vi "FPGAcode4_SmallArray.vi"() -> ()   [LabVIEW 2015]
uses:
  Limits_In.ctl
  Detector_Cluster.ctl
  <vilib>/Platform/TimedLoop/XDataNode/timing_clust.ctl
  <vilib>/Platform/TimedLoop/XDataNode/nitl_modes.ctl
  <vilib>/Platform/TimedLoop/XDataNode/wakeup.ctl
  Correlations.ctl
  <vilib>/rvi/Emulation/niFpgaSctlEmulationGetInTimedLoop.vi
  <vilib>/rvi/Emulation/niFpgaEmulationReportErrorSimple.vi
  <vilib>/rvi/Emulation/niFpgaGetClockAttributes.vi
  <vilib>/rvi/Emulation/niFpgaCriticalErrorInLSC.vi
  <vilib>/rvi/eio/common/nirviEmuTemplateMethod_errors.vi
  <vilib>/rvi/Emulation/niFpgaEmulationIsFPGAContextNoSignature.vi
  <vilib>/rvi/DataTransferAndStorage/Container/Common/niFpgaContainerGetUniqueNameForEmu.vi
  <vilib>/rvi/eio/common/nirviEmuReportErrorAndStop.vi
  <vilib>/rvi/Emulation/niFpgaProcessEmulError.vi
  <vilib>/Platform/TimedLoop/XDataNode/XDataNode.xnode
  <vilib>/eio/EIONode/EIONode.xnode
  <vilib>/rvi/DataTransferAndStorage/Container/XNode/niFpgaContainer.xnode
  <vilib>/rvi/DataTransferAndStorage/Handshake/Emulation/niFpgaHandshakeEmulation.vi
  <vilib>/Platform/TimedLoop/XDataNode/XDNodeRunTimeDep.lvlib
panel:
  in  "Charge Error Factor":fxp<+,32,0>=0.19999999995343387 format="%_2g"
  in  "Calibrate":bool=TRUE
  in  "Limits":T1={"High Charge Limit"=4.54747350780585e-13, "Low Charge Limit"=0.0, "High Velocity Limit"=262143.0, "Low Velocity Limit"=0.0, "High Mass Limit"=7.27595761248936e-12, "Low Mass Limit"=0.0, "High Voltage"=2200000.0}
  in  "One Shot":bool
  in  "Threshold Factor":fxp<+/-,32,16>=1.149993896484375 format="%.2g"
  in  "Armed":bool
  in  "User Trigger Distance":fxp<+/-,34,18> format="%.3g"
  in  "User Trigger?":bool
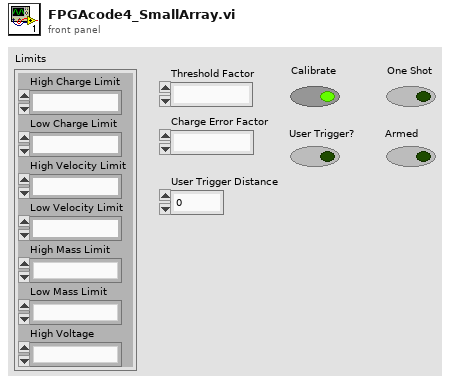
[diagram p1: front panel]
types:
  T1 = typedef "Limits_In.ctl" = cluster{"High Charge Limit":fxp<+,32,-41>, "Low Charge Limit":fxp<+,32,-41>, "High Velocity Limit":fxp<+,18,18>, "Low Velocity Limit":fxp<+,18,18>, "High Mass Limit":fxp<+,32,-37>, "Low Mass Limit":fxp<+,32,-37>, "High Voltage":fxp<+,32,22>}
  T2 = cluster{"[0]":fxp<+,16,1>, "[1]":fxp<+,16,1>, "[2]":fxp<+,16,1>, "[3]":fxp<+,16,1>, "[4]":fxp<+,16,1>, "[5]":fxp<+,16,1>, "[6]":fxp<+,16,1>, "[7]":fxp<+,16,1>, "[8]":fxp<+,16,1>, "[9]":fxp<+,16,1>, "[10]":fxp<+,16,1>}
  T3 = cluster{"[0]":i32, "[1]":i32, "[2]":i32, "[3]":i32, "[4]":i32, "[5]":i32, "[6]":i32, "[7]":i32, "[8]":i32, "[9]":i32, "[10]":i32}
  T4 = cluster{"[0]":cluster{"Detector Max Speed Count":i32, "Detector Min Speed Count":i32, "Gap Max Speed Count":i32, "Gap Min Speed Count":i32}, "[1]":cluster{"Detector Max Speed Count":i32, "Detector Min Speed Count":i32, "Gap Max Speed Count":i32, "Gap Min Speed Count":i32}, "[2]":cluster{"Detector Max Speed Count":i32, "Detector Min Speed Count":i32, "Gap Max Speed Count":i32, "Gap Min Speed Count":i32}, "[3]":cluster{"Detector Max Speed Count":i32, "Detector Min Speed Count":i32, "Gap Max Speed Count":i32, "Gap Min Speed Count":i32}, "[4]":cluster{"Detector Max Speed Count":i32, "Detector Min Speed Count":i32, "Gap Max Speed Count":i32, "Gap Min Speed Count":i32}, "[5]":cluster{"Detector Max Speed Count":i32, "Detector Min Speed Count":i32, "Gap Max Speed Count":i32, "Gap Min Speed Count":i32}, "[6]":cluster{"Detector Max Speed Count":i32, "Detector Min Speed Count":i32, "Gap Max Speed Count":i32, "Gap Min Speed Count":i32}, "[7]":cluster{"Detector Max Speed Count":i32, "Detector Min Speed Count":i32, "Gap Max Speed Count":i32, "Gap Min Speed Count":i32}, "[8]":cluster{"Detector Max Speed Count":i32, "Detector Min Speed Count":i32, "Gap Max Speed Count":i32, "Gap Min Speed Count":i32}, "[9]":cluster{"Detector Max Speed Count":i32, "Detector Min Speed Count":i32, "Gap Max Speed Count":i32, "Gap Min Speed Count":i32}, "[10]":cluster{"Detector Max Speed Count":i32, "Detector Min Speed Count":i32, "Gap Max Speed Count":i32, "Gap Min Speed Count":i32}}
  T5 = cluster{cluster{"[0]":i32, "[1]":i32, "[2]":i32, "[3]":i32, "[4]":i32, "[5]":i32, "[6]":i32, "[7]":i32, "[8]":i32, "[9]":i32, "[10]":i32}, cluster{"[0]":i32, "[1]":i32, "[2]":i32, "[3]":i32, "[4]":i32, "[5]":i32, "[6]":i32, "[7]":i32, "[8]":i32, "[9]":i32, "[10]":i32}, cluster{"[0]":i32, "[1]":i32, "[2]":i32, "[3]":i32, "[4]":i32, "[5]":i32, "[6]":i32, "[7]":i32, "[8]":i32, "[9]":i32, "[10]":i32}, cluster{"[0]":i32, "[1]":i32, "[2]":i32, "[3]":i32, "[4]":i32, "[5]":i32, "[6]":i32, "[7]":i32, "[8]":i32, "[9]":i32, "[10]":i32}}
  T6 = cluster{"Distance to PSU":fxp<+/-,64,37>, "Distance to end of PSU":fxp<+/-,64,37>, "Distance to DCS 2":fxp<+/-,64,37>, "Distance to DCS 1":fxp<+/-,64,37>, "Distance to front of LEIL Chamber":fxp<+/-,64,37>}
  T7 = typedef "Detector_Cluster.ctl" = cluster{"Det 1":i32, "Det 2":i32}
  T8 = cluster{"Filter 1":T7, "Filter 2":T7, "Filter 3":T7, "Filter 4":T7}
  T9 = cluster{"Detector Max Speed Count":i32, "Detector Min Speed Count":i32, "Gap Max Speed Count":i32, "Gap Min Speed Count":i32}[]
  T10 = cluster{"Filter 1":T7, "Filter 2":T7, "Filter 3":T7, "Filter 4":T7}[]
  T11 = typedef "XDNodeRunTimeDep.lvlib/timing_clust.ctl" = cluster{"Expected End [f-1]":u64, "Actual End [f-1]":u64, "Finished Late? [f-1]":bool, "Expected End [i-1]":u64, "Actual End [i-1]":u64, "Finished Late? [i-1]":bool, "Expected Start [i]":u64, "Actual Start [i]":u64, "Expected Start [f]":u64, "Actual Start [f]":u64, "Source Name":string, "Structure Name":string, "Period":i64, "Deadline":i64, "Offset":i64, "Start":i64, "Priority":i32, "Timeout":i32, "Mode":T12, "Wakeup Reason":T13, "Error":errorcluster, "Source Type":string, "Secondary Source Type":string, "Global End Time":u64, "Global Start Time":u64, "Frame Duration":u64, "Iteration Duration":u64, "Assigned CPU":i32, "I/O Scan Engine Mode":u32}
  T12 = typedef "XDNodeRunTimeDep.lvlib/nitl_modes.ctl" = enum32{"No Change", "Process missed periods, maintain original phase", "Discard missed periods, maintain original phase", "Process missed periods, ignore original phase", "Discard missed periods, ignore original phase"}
  T13 = typedef "XDNodeRunTimeDep.lvlib/wakeup.ctl" = enum32{"Normal", "Aborted", "Asynchronous wakeup", "Timing source error", "Timed loop error", "Timeout"}
  T14 = cluster{"IO Module\\AI 0":i16, "IO Module\\AI 1":i16}
  T15 = cluster{"First Detector Count":i32, "Detector Gap Count":i32, "Second Detector Count":i32, "Second Detector Final Count":i32}
  T16 = typedef "Correlations.ctl" = cluster{"First Correlation":i32, "Latest Correlation":i32}
  T17 = cluster{"Data":fxp<+/-,40,32>, "Data":fxp<+/-,40,32>}
  T18 = cluster{cluster{"Data":i16, "Data":i16}, cluster{"Det 1":i16, "Det 2":i16}, cluster{"Det 1":i16, "Det 2":i16}, cluster{"Det 1":i16, "Det 2":i16}}
  T19 = cluster{cluster{"Det 1":i16, "Det 2":i16}, cluster{"Det 1":i16, "Det 2":i16}, cluster{"Det 1":i16, "Det 2":i16}, cluster{"Det 1":i16, "Det 2":i16}}
  T20 = cluster{"Distance to PSU":fxp<+/-,64,69>, "Distance to end of PSU":fxp<+/-,64,69>, "Distance to DCS 2":fxp<+/-,64,69>, "Distance to DCS 1":fxp<+/-,64,69>, "Distance to front of LEIL Chamber":fxp<+/-,64,69>}
  T21 = cluster{"Distance to PSU":i32, "Distance to end of PSU":i32, "Distance to DCS 2":i32, "Distance to DCS 1":i32, "Distance to front of LEIL Chamber":i32}
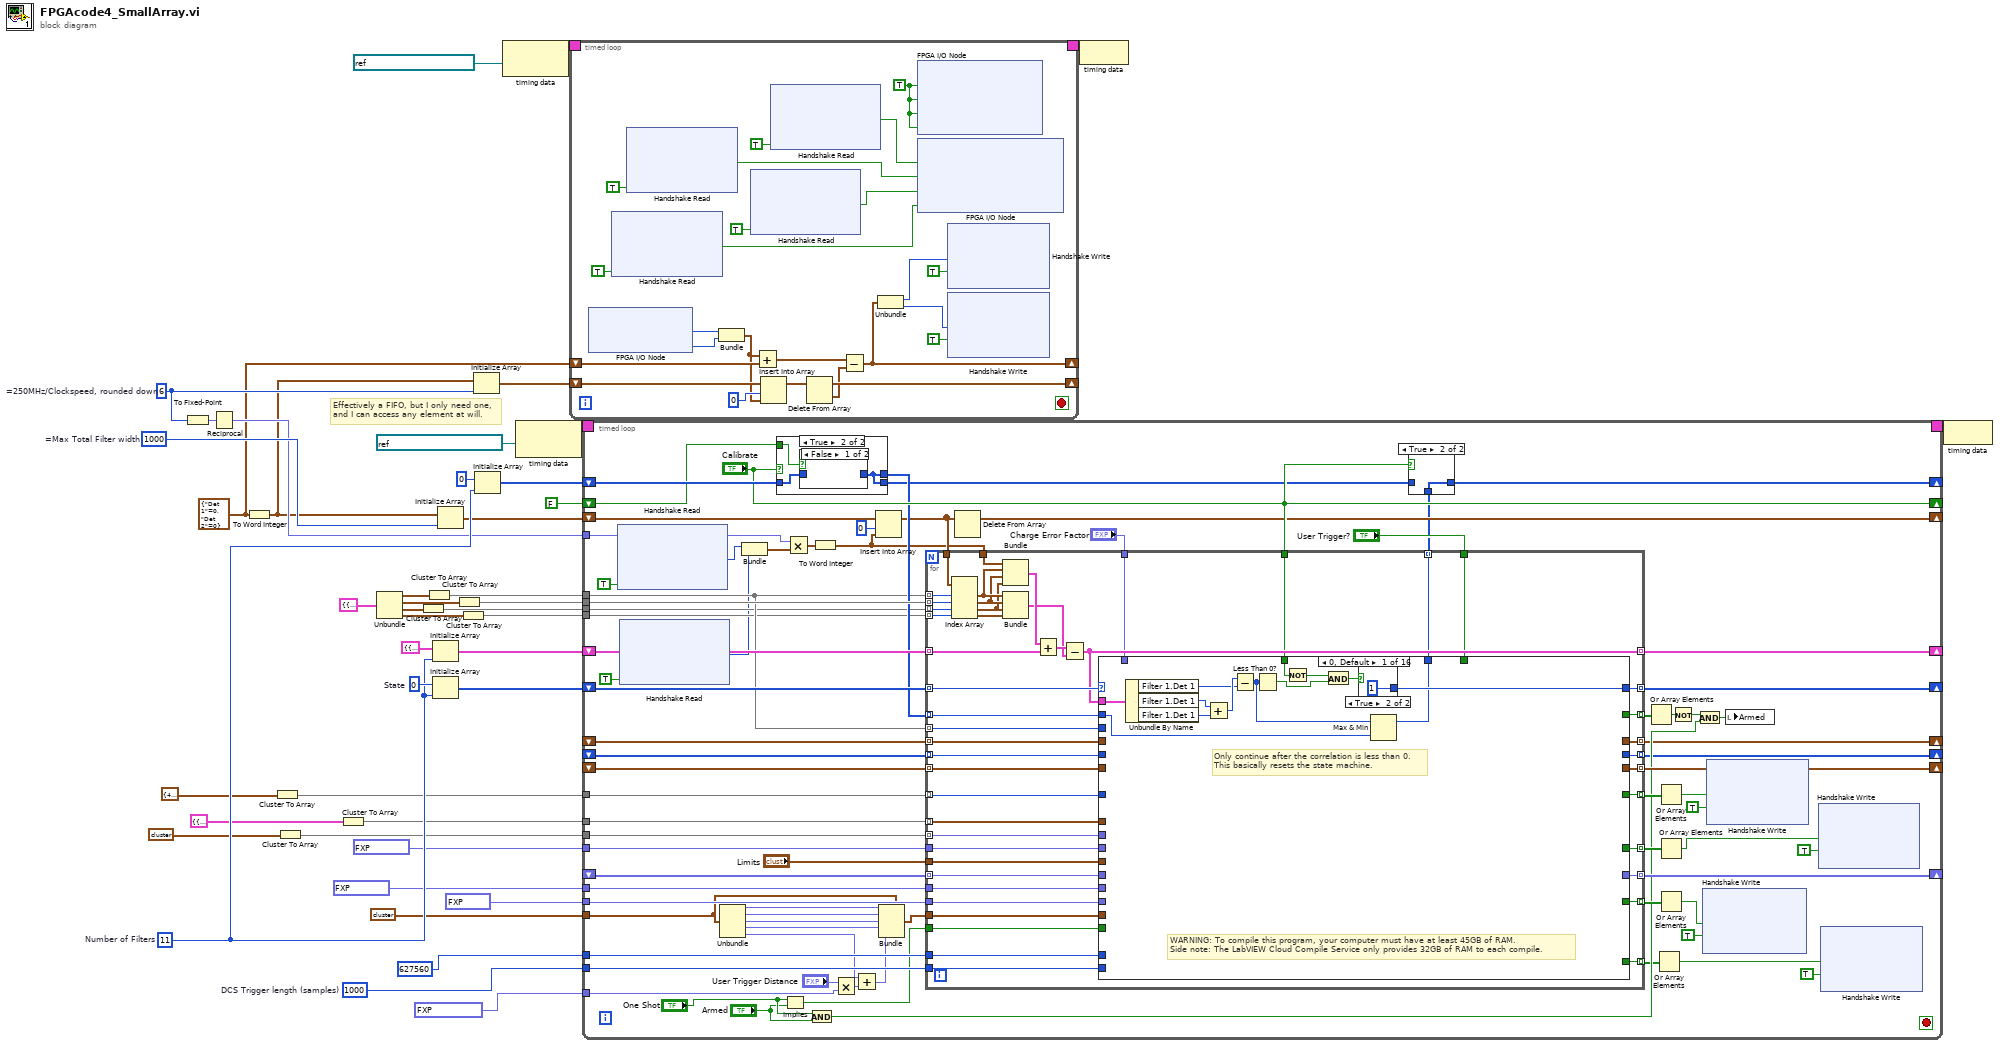
[diagram p0: block diagram]
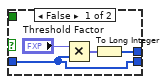
[diagram p2: hidden frame]
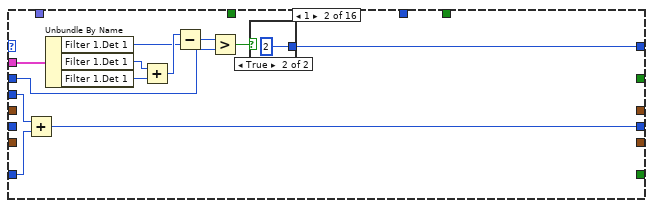
[diagram p6: hidden frame]
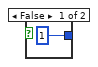
[diagram p7: hidden frame]
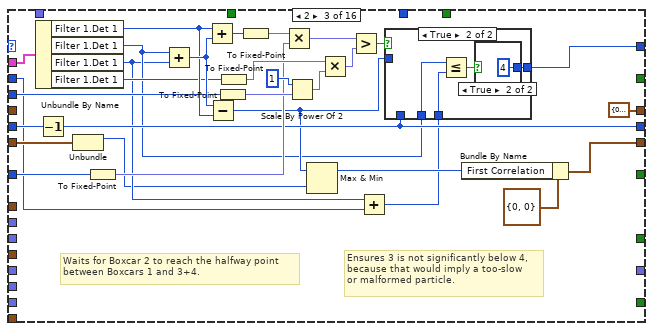
[diagram p8: hidden frame]
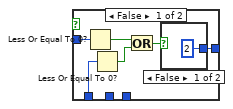
[diagram p9: hidden frame]
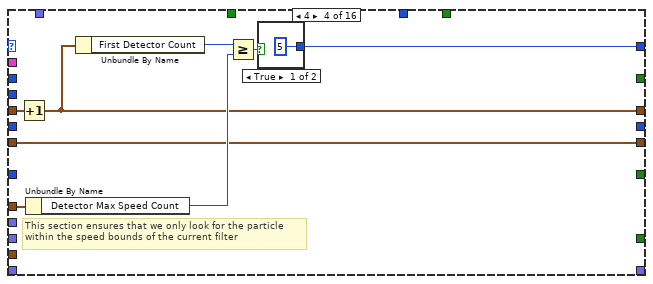
[diagram p12: hidden frame]
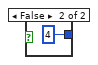
[diagram p13: hidden frame]
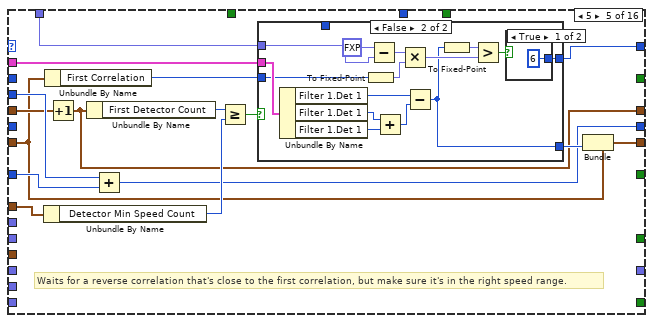
[diagram p14: hidden frame]
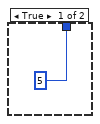
[diagram p15: hidden frame]
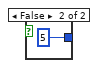
[diagram p16: hidden frame]
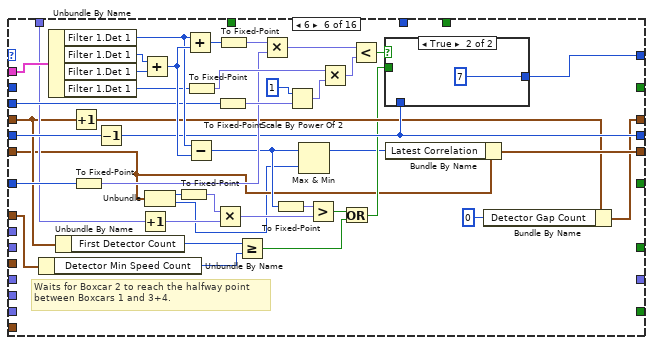
[diagram p17: hidden frame]
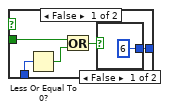
[diagram p18: hidden frame]
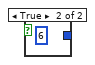
[diagram p19: hidden frame]
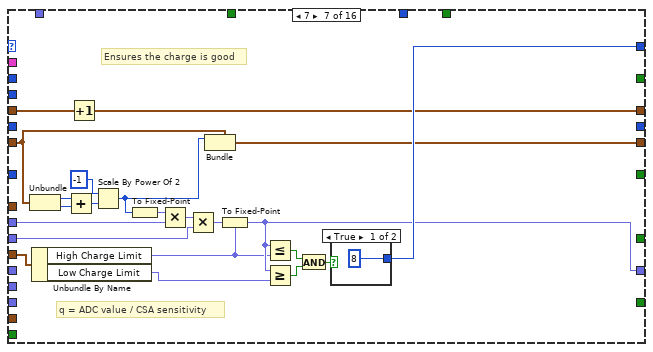
[diagram p20: hidden frame]
diagram:
  w35 = u8 6  # =250MHz/Clockspeed, rounded down
  w40 = 1000  # =Max Total Filter width
  w5 = u16 1000  # DCS Trigger length (samples)
  w2 = T7 {"Det 1"=0, "Det 2"=0} ("Detectors")
  w44 = u8 0  # State
  w41 = 11  # Number of Filters
  # "Effectively a FIFO, but I only need one,\nand I can access any element at will."
  n1 = To Fixed-Point(number=w35) -> (fixed-point=w37:fxp<+,8,8>)  [unwired: 1 in]
  n2 = Reciprocal(x=w37) -> (1/x=w20:fxp<+,9,1>)
  n3 = To Word Integer(number=w2) -> (16bit integer=w1:cluster{"Det 1":i16, "Det 2":i16})
  n4 = Cluster To Array(cluster=T3 {"[0]"=4000, "[1]"=2359, "[2]"=1391, "[3]"=820, "[4]"=484, "[5]"=285, "[6]"=168, "[7]"=99, "[8]"=59, "[9]"=35, "[10]"=20}) -> (array=w13:i32[])
  n5 = Cluster To Array(cluster=T2 {"[0]"=0.000823974609375, "[1]"=0.000823974609375, "[2]"=0.000823974609375, "[3]"=0.000823974609375, "[4]"=0.000823974609375, "[5]"=0.00152587890625, "[6]"=0.003265380859375, "[7]"=0.007080078125, "[8]"=0.015869140625, "[9]"=0.03704833984375, "[10]"=0.100006103515625} ("cluster 3")) -> (array=w11:fxp<+,16,1>[])
  n6 = Cluster To Array(cluster=T4 {"[0]"={"Detector Max Speed Count"=42000, "Detector Min Speed Count"=84000, "Gap Max Speed Count"=78000, "Gap Min Speed Count"=156000}, "[1]"={"Detector Max Speed Count"=21477, "Detector Min Speed Count"=42953, "Gap Max Speed Count"=39885, "Gap Min Speed Count"=79770}, "[2]"={"Detector Max Speed Count"=10982, "Detector Min Speed Count"=21964, "Gap Max Speed Count"=20395, "Gap Min Speed Count"=40790}, "[3]"={"Detector Max Speed Count"=5616, "Detector Min Speed Count"=11231, "Gap Max Speed Count"=10429, "Gap Min Speed Count"=20858}, "[4]"={"Detector Max Speed Count"=2872, "Detector Min Speed Count"=5743, "Gap Max Speed Count"=5333, "Gap Min Speed Count"=10666}, "[5]"={"Detector Max Speed Count"=1468, "Detector Min Speed Count"=2937, "Gap Max Speed Count"=2727, "Gap Min Speed Count"=5454}, "[6]"={"Detector Max Speed Count"=751, "Detector Min Speed Count"=1502, "Gap Max Speed Count"=1394, "Gap Min Speed Count"=2789}, "[7]"={"Detector Max Speed Count"=384, "Detector Min Speed Count"=768, "Gap Max Speed Count"=713, "Gap Min Speed Count"=1426}, "[8]"={"Detector Max Speed Count"=196, "Detector Min Speed Count"=393, "Gap Max Speed Count"=365, "Gap Min Speed Count"=729}, "[9]"={"Detector Max Speed Count"=100, "Detector Min Speed Count"=201, "Gap Max Speed Count"=186, "Gap Min Speed Count"=373}, "[10]"={"Detector Max Speed Count"=51, "Detector Min Speed Count"=103, "Gap Max Speed Count"=95, "Gap Min Speed Count"=191}} ("cluster 2")) -> (array=w12:T9)
  n7 = Unbundle(T5 {{"[0]"=1200, "[1]"=1200, "[2]"=1200, "[3]"=1200, "[4]"=1200, "[5]"=650, "[6]"=306, "[7]"=140, "[8]"=62, "[9]"=26, "[10]"=10}, {"[0]"=5200, "[1]"=3559, "[2]"=2591, "[3]"=2020, "[4]"=1684, "[5]"=935, "[6]"=474, "[7]"=240, "[8]"=122, "[9]"=62, "[10]"=30}, {"[0]"=5800, "[1]"=4159, "[2]"=3191, "[3]"=2620, "[4]"=2284, "[5]"=1260, "[6]"=627, "[7]"=310, "[8]"=153, "[9]"=75, "[10]"=35}, {"[0]"=6400, "[1]"=4759, "[2]"=3791, "[3]"=3220, "[4]"=2884, "[5]"=1585, "[6]"=780, "[7]"=380, "[8]"=184, "[9]"=88, "[10]"=40}} ("output cluster")) -> (w33:T3, w32:T3, w31:T3, w30:T3)
  n8 = Cluster To Array(cluster=w31) -> (array=w17:i32[])
  n9 = Cluster To Array(cluster=w33) -> (array=w19:i32[])
  n10 = Initialize Array(T8 {"Filter 1"={"Det 1"=0, "Det 2"=0}, "Filter 2"={"Det 1"=0, "Det 2"=0}, "Filter 3"={"Det 1"=0, "Det 2"=0}, "Filter 4"={"Det 1"=0, "Det 2"=0}} ("cluster"), w41) -> (w15:T10)
  n11 = Initialize Array(w44, w41) -> (w14:u8[])
  n12 = Initialize Array(w1, w40) -> (w21:cluster{"Det 1":i16, "Det 2":i16}[])
  n13 = Cluster To Array(cluster=w32) -> (array=w18:i32[])
  n14 = Cluster To Array(cluster=w30) -> (array=w16:i32[])
  n15 = Initialize Array(w1, w35) -> (w36:cluster{"Det 1":i16, "Det 2":i16}[])
  n16 = Initialize Array(0 ("Thresholds in"), w41) -> (w22:i32[])
  n17 = node-c288(refnum<k21> "IO Module\\Data Clock" ("Source Name")) -> (w39:T11)
  n18 = node-c288(refnum<k21> "40 MHz Onboard Clock" ("Source Name")) -> (w25:T11)
  n19 = timed-loop {
    timing: w39 -> [_]
    timing-out: [_] -> w38
    shift-right: [w58] -> _
    shift-left: w2 -> [w67]
    shift-right: [w60] -> _
    shift-left: w36 -> [w65]
    stop <- _ stop-if-true
    w45 = TRUE ("IO Module\\PFI Enable")
    n20 = xnode "FPGA I/O Node"() -> ("IO Module\\AI 0"=w64:i16, "IO Module\\AI 1"=w63:i16)  [unwired: 2 in, 2 out]
    n21 = xnode ("Handshake Read")("Ready for Output"=TRUE) -> ("Data"=w53:bool)  [unwired: 1 in, 2 out]
    n22 = xnode ("Handshake Read")("Ready for Output"=TRUE) -> ("Data"=w49:bool)  [unwired: 1 in, 2 out]
    n23 = Bundle("IO Module\\AI 0"=w64, "IO Module\\AI 1"=w63) -> (w62:T14)  [unwired: 1 in]
    n24 = xnode ("Handshake Read")("Ready for Output"=TRUE) -> ("Data"=w52:bool)  [unwired: 1 in, 2 out]
    n25 = Add(x=w62, y=w67) -> (x+y=w66:T7)
    n26 = Insert Into Array(array=w65, index=0, new element=w62) -> (w61:cluster{"Det 1":i16, "Det 2":i16}[])
    n27 = xnode ("Handshake Read")("Ready for Output"=TRUE) -> ("Data"=w46:bool)  [unwired: 1 in, 2 out]
    n28 = Delete From Array(array=w61) -> (deleted portion=w59:cluster{"Det 1":i16, "Det 2":i16}, array with subset deleted=w60:cluster{"Det 1":i16, "Det 2":i16}[])  [unwired: 2 in]
    n29 = Subtract(x=w66, y=w59) -> (x-y=w58:T7)
    n30 = Unbundle(w58) -> ("Det 1"=w56:i32, "Det 2"=w54:i32)
    n31 = xnode "FPGA I/O Node"("IO Module\\PFI 0 WE"=w45, "IO Module\\PFI 1 WE"=w45, "IO Module\\PFI 2 WE"=w45, "IO Module\\PFI 3 WE"=w45) -> ()  [unwired: 4 in, 4 out]
    n32 = xnode "FPGA I/O Node"("IO Module\\PFI 0 Wr Data"=w46, "IO Module\\PFI 1 Wr Data"=w49, "IO Module\\PFI 2 Wr Data"=w52, "IO Module\\PFI 3 Wr Data"=w53) -> ()  [unwired: 4 in, 4 out]
    n33 = xnode ("Handshake Write")("Data"=w56, "Input Valid"=TRUE) -> ()  [unwired: 1 in, 2 out]
    n34 = xnode ("Handshake Write")("Data"=w54, "Input Valid"=TRUE) -> ()  [unwired: 1 in, 2 out]
  }
  n35 = timed-loop {
    shift-right: [w89] -> _
    shift-left: w21 -> [w147]
    shift-right: [w97] -> _
    shift-left: w15 -> [w144]
    shift-right: [w91] -> _
    shift-left: w14 -> [w146]
    shift-right: [w98] -> _
    shift-left: _ -> [w145]
    tunnel: w12 -> [w143]
    shift-right: [w142] -> _
    shift-left: _ -> [w141]
    tunnel: w19 -> [w96]
    tunnel: w18 -> [w140]
    tunnel: w13 -> [w139]
    tunnel: w11 -> [w138]
    shift-right: [w137] -> _
    shift-left: _ -> [w136]
    tunnel: fxp<+,32,-43> 9.525990075777386e-16 ("fixed-point 2") -> [w135]
    tunnel: fxp<+,32,-49> 2.2727300016438096e-16 ("fixed-point 3") -> [w134]
    tunnel: fxp<+,28,28> 32400000.0 ("fixed-point") -> [w133]
    tunnel: T6 {"Distance to PSU"=1.2345678955316544, "Distance to end of PSU"=2.4691357985138893, "Distance to DCS 2"=3.229876533150673, "Distance to DCS 1"=-1.677654318511486, "Distance to front of LEIL Chamber"=5.305777758359909} ("x/y") -> [w126]
    shift-right: [w132] -> _
    shift-left: w22 -> [w131]
    shift-right: ["Calibrate"] -> _
    shift-left: FALSE ("Calibrate") -> [w130]
    tunnel: w5 -> [w129]
    tunnel: 627560 ("32bit integer") -> [w128]
    tunnel: fxp<+,32,1> 1.2345679011195898 ("1/x") -> [w127]
    shift-right: [w95] -> _
    shift-left: _ -> [w94]
    tunnel: w16 -> [w93]
    tunnel: w17 -> [w92]
    timing: w25 -> [_]
    timing-out: [_] -> w24
    tunnel: w20 -> [w87]
    stop <- _ stop-if-true
    n36 = xnode ("Handshake Read")("Ready for Output"=TRUE) -> ("Data"=w74:i32)  [unwired: 1 in, 2 out]
    n37 = xnode ("Handshake Read")("Ready for Output"=TRUE) -> ("Data"=w73:i32)  [unwired: 1 in, 2 out]
    n38 = Unbundle(w126) -> ("Distance to PSU"=w120:fxp<+/-,64,37>, "Distance to end of PSU"=w119:fxp<+/-,64,37>, "Distance to DCS 2"=w118:fxp<+/-,64,37>, "Distance to DCS 1"=w115:fxp<+/-,64,37>, "Distance to front of LEIL Chamber"=w114:fxp<+/-,64,37>)
    n39 = Bundle("Data"=w74, "Data"=w73) -> (w72:cluster{"Data":i32, "Data":i32})  [unwired: 1 in]
    n40 = case shown="True" "Calibrate" {
      tunnel: w131 -> [w149 w153]
      tunnel: [w149 w152] -> w99
      tunnel: w130 -> [_ w154]
      tunnel: [w148 w152] -> w100
      frame False {
        n41 = Multiply(x="Threshold Factor", y=w149) -> (x*y=w150:fxp<+/-,64,48>[])
        n42 = To Long Integer(number=w150) -> (32bit integer=w148:i32[])
      }
      frame True {
        n43 = case shown="False" w154 {
          tunnel: w153 -> [_ w155]
          tunnel: [_ w155] -> w152
          frame False {
          }
          frame True {
          }
        }
      }
    }
    n44 = Implies(1:"Armed", 2:"One Shot") -> (0:w122:bool)
    n45 = Multiply(x=w87, y=w72) -> (x*y=w88:T17)
    n46 = And(x="One Shot", y="Armed") -> (x .and. y?=w106:bool)
    n47 = To Word Integer(number=w88) -> (16bit integer=w86:cluster{"Data":i16, "Data":i16})
    n48 = Multiply(x="User Trigger Distance", y=w127) -> (x*y=w116:fxp<+/-,64,18>)
    n49 = Add(x=w114, y=w116) -> (x+y=w113:fxp<+/-,64,38>)
    n50 = Insert Into Array(array=w147, index=0, new element=w86) -> (w90:cluster{"Det 1":i16, "Det 2":i16}[])
    n51 = Bundle(cluster=w126, "Distance to PSU"=w120, "Distance to end of PSU"=w119, "Distance to DCS 2"=w118, "Distance to DCS 1"=w115, "Distance to front of LEIL Chamber"=w113) -> (w117:T6)
    n52 = for {
      tunnel: w90 -> [w204]
      tunnel: [w190] -> w97 mode=indexing
      tunnel: w146 -> [w203] mode=indexing
      tunnel: [w202] -> w91 mode=indexing
      tunnel: w100 -> [w163] mode=indexing
      tunnel: [w201] -> w98 mode=indexing
      tunnel: w145 -> [w200] mode=indexing
      tunnel: w144 -> [w194] mode=indexing
      tunnel: w86 -> [w199]
      tunnel: w143 -> [w189] mode=indexing
      tunnel: [w188] -> w142 mode=indexing
      tunnel: w141 -> [w187] mode=indexing
      tunnel: w96 -> [w186] mode=indexing
      tunnel: w140 -> [w161] mode=indexing
      tunnel: w92 -> [w185] mode=indexing
      tunnel: w93 -> [w184] mode=indexing
      tunnel: w96 -> [w165] mode=indexing
      tunnel: w139 -> [w164] mode=indexing
      tunnel: "Charge Error Factor" -> [w183]
      tunnel: w138 -> [w182] mode=indexing
      tunnel: "Limits" -> [w181]
      tunnel: [w180] -> w137 mode=indexing
      tunnel: w136 -> [w179] mode=indexing
      tunnel: w135 -> [w178]
      tunnel: w134 -> [w177]
      tunnel: w133 -> [w176]
      tunnel: w117 -> [w175]
      tunnel: w122 -> [w174]
      tunnel: w129 -> [w172]
      tunnel: w128 -> [w173]
      tunnel: [w171] -> w112 mode=indexing
      tunnel: [w170] -> w111 mode=indexing
      tunnel: [w169] -> w110 mode=indexing
      tunnel: [w168] -> w109 mode=indexing
      tunnel: "User Trigger?" -> [w167]
      tunnel: "Calibrate" -> [w166]
      tunnel: [w162] -> w95 mode=indexing
      tunnel: w94 -> [w160] mode=indexing
      tunnel: [w159] -> w85 mode=indexing
      tunnel: [w158] -> w71 mode=indexing
      n53 = Index Array(array=w204, index #1=w186, index #2=w161, index #3=w185, index #4=w184) -> (element #1=w197:cluster{"Det 1":i16, "Det 2":i16}, element #2=w196:cluster{"Det 1":i16, "Det 2":i16}, element #3=w195:cluster{"Det 1":i16, "Det 2":i16}, element #4=w198:cluster{"Det 1":i16, "Det 2":i16})
      n54 = Bundle(w199, w197, w196, w195) -> (w193:T18)  [unwired: 1 in]
      n55 = Bundle(w197, w196, w195, w198) -> (w191:T19)  [unwired: 1 in]
      n56 = Add(x=w193, y=w194) -> (x+y=w192:T8)
      n57 = Subtract(x=w192, y=w191) -> (x-y=w190:T8)
      n58 = case shown="0, Default" w203 {
        tunnel: w163 -> [w207 w230 w236 _ _ _ _ _ _ _ _ _ _ _ _ _]
        tunnel: [w216 w229 w261 w278 w293 w359 w381 w395 w409 w472 w485 w499 w560 w587 u8 16 ("Det 3") w651] -> w202
        tunnel: w165 -> [_ w222 w255 _ w295 w351 _ _ w411 w464 _ w501 w552 _ w619 _]
        tunnel: [_ _ T15 {"First Detector Count"=0, "Detector Gap Count"=0, "Second Detector Count"=0, "Second Detector Final Count"=0} ("Cutoffs") w275 w285 w322 w371 w392 w403 w436 w482 w494 w540 w570 w610 w649] -> w201
        tunnel: w200 -> [_ _ _ w276 w290 w327 w372 w393 w406 w442 w483 w496 w530 w570 w609 w650]
        tunnel: w160 -> [_ _ w262 _ _ w360 _ _ _ w473 _ _ w561 _ _ w632]
        tunnel: w190 -> [w211 w224 w248 _ w296 w344 _ _ w412 w458 _ w502 w546 _ _ _]
        tunnel: w189 -> [_ _ _ w282 w300 w328 _ w399 w416 w441 w489 w506 w531 _ _ _]
        tunnel: w187 -> [_ _ w239 w277 w287 w326 w374 w394 w405 w451 w484 w492 w524 _ _ _]
        tunnel: w164 -> [_ w221 w256 _ w294 w352 _ _ w410 w465 _ w500 w553 _ w613 _]
        tunnel: w183 -> [_ _ _ _ w297 w337 _ _ w413 w452 _ w503 w539 _ _ _]
        tunnel: w182 -> [_ _ _ _ _ _ w386 _ _ _ _ _ _ _ _ _]
        tunnel: w181 -> [_ _ _ _ _ _ w389 _ _ _ _ _ _ w598 _ _]
        tunnel: [_ _ _ _ _ _ w369 w391 w402 w434 w481 w493 w525 _ _ _] -> w180
        tunnel: w179 -> [_ _ _ _ _ _ _ w391 w402 w434 w481 w493 w525 w576 _ _]
        tunnel: w178 -> [_ _ _ _ _ _ _ _ _ _ _ _ _ w597 _ _]
        tunnel: w177 -> [_ _ _ _ _ _ w379 _ _ _ _ _ _ _ _ _]
        tunnel: w176 -> [_ _ _ _ _ _ _ _ _ _ _ _ _ w575 _ _]
        tunnel: w175 -> [_ _ _ _ _ _ _ _ _ _ _ _ _ _ w622 _]
        tunnel: w174 -> [_ _ _ _ _ _ _ _ _ _ _ _ _ w581 _ _]
        tunnel: w173 -> [_ _ _ _ _ _ _ _ _ _ _ _ _ _ w616 _]
        tunnel: w172 -> [_ _ _ _ _ _ _ _ _ _ _ _ _ _ _ w629]
        tunnel: [_ _ _ _ _ _ _ _ _ _ _ _ _ _ _ w648] -> w171
        tunnel: [_ _ _ _ _ _ _ _ _ _ _ _ _ _ _ w647] -> w170
        tunnel: [_ _ _ _ _ _ _ _ _ _ _ _ _ _ _ w631] -> w169
        tunnel: [_ _ _ _ _ _ _ _ _ _ _ _ _ w580 _ _] -> w168
        tunnel: w167 -> [_ _ _ _ _ _ _ _ _ _ _ _ _ _ _ w633]
        tunnel: w166 -> [w209 _ _ _ _ _ _ _ _ _ _ _ _ _ _ _]
        tunnel: [_ w220 w244 _ w286 w340 _ _ w404 w454 _ w495 w542 _ _ w625] -> w162
        tunnel: [_ _ w250 w277 w289 w346 w373 w394 w405 w451 w484 w492 w524 _ _ _] -> w188
        tunnel: [w205 _ _ _ _ _ _ _ _ _ _ _ _ _ _ _] -> w159
        tunnel: [_ _ _ _ _ _ _ _ _ _ _ _ _ _ _ w630] -> w158
        frame 0, Default {
          # "WARNING: To compile this program, your computer must have at least 45GB of RAM.\nSide note: The LabVIEW Cloud Compile Service only provides 32GB of RAM to each compile."
          # "Only continue after the correlation is less than 0.\nThis basically resets the state machine."
          n59 = Unbundle By Name(w211) -> ("Filter 1.Det 1"=w212:i32, "Filter 1.Det 1"=w213:i32, "Filter 1.Det 1"=w214:i32)
          n60 = Add(x=w213, y=w214) -> (x+y=w215:i32)
          n61 = Subtract(x=w215, y=w212) -> (x-y=w206:i32)
          n62 = Less Than 0?(x=w206) -> (x < 0?=w217:bool)
          n63 = Not(x=w209) -> (.not. x?=w208:bool)
          n64 = And(x=w208, y=w217) -> (x .and. y?=w210:bool)
          n65 = case shown="True" w210 {
            tunnel: [_ u8 1 ("Det 3")] -> w216
            frame False {
            }
            frame True {
            }
          }
          n66 = Max & Min(x=w206, y=w207) -> (max(x,y)=w205:i32)  [unwired: 1 out]
        }
        frame 1 {
          n67 = Add(x=w222, y=w221) -> (x+y=w220:i32)
          n68 = Unbundle By Name(w224) -> ("Filter 1.Det 1"=w225:i32, "Filter 1.Det 1"=w226:i32, "Filter 1.Det 1"=w227:i32)
          n69 = Add(x=w226, y=w227) -> (x+y=w228:i32)
          n70 = Subtract(x=w228, y=w225) -> (x-y=w223:i32)
          n71 = Greater?(x=w223, y=w230) -> (0:w219:bool)
          n72 = case shown="True" w219 {
            tunnel: [u8 1 ("Det 3") u8 2 ("Det 3")] -> w229
            frame False {
            }
            frame True {
            }
          }
        }
        frame 2 {
          # "Ensures 3 is not significantly below 4,\nbecause that would imply a too-slow\nor malformed particle."
          # "Waits for Boxcar 2 to reach the halfway point\nbetween Boxcars 1 and 3+4."
          n73 = Unbundle By Name(w248) -> ("Filter 1.Det 1"=w258:i32, "Filter 1.Det 1"=w235:i32, "Filter 1.Det 1"=w234:i32, "Filter 1.Det 1"=w252:i32)
          n74 = Decrement(x=w262) -> (x-1=w244:i32)
          n75 = Unbundle(w239) -> ("First Correlation"=w233:i32)  [unwired: 1 out]
          n76 = To Fixed-Point(number=w256) -> (fixed-point=w245:fxp<+/-,32,32>)  [unwired: 1 in]
          n77 = Add(x=w235, y=w234) -> (x+y=w259:i32)
          n78 = Add(x=w258, y=w259) -> (x+y=w260:i32)
          n79 = Subtract(x=w259, y=w258) -> (x-y=w240:i32)
          n80 = To Fixed-Point(number=w255) -> (fixed-point=w246:fxp<+/-,32,32>)  [unwired: 1 in]
          n81 = To Fixed-Point(number=w252) -> (fixed-point=w247:fxp<+/-,32,32>)  [unwired: 1 in]
          n82 = To Fixed-Point(number=w260) -> (fixed-point=w249:fxp<+/-,32,32>)  [unwired: 1 in]
          n83 = Multiply(x=w249, y=w245) -> (x*y=w257:fxp<+/-,64,64>)
          n84 = Scale By Power Of 2(n=i16 1, x=w246) -> (x*2^n=w253:fxp<+/-,32,32>)
          n85 = Max & Min(x=w240, y=w233) -> (max(x,y)=w241:i32)  [unwired: 1 out]
          n86 = Multiply(x=w247, y=w253) -> (x*y=w251:fxp<+/-,64,64>)
          n87 = Greater?(x=w257, y=w251) -> (0:w242:bool)
          n88 = Add(x=w234, y=w236) -> (x+y=w237:i32)
          n89 = case shown="True" w242 {
            tunnel: [w268 w273] -> w261
            tunnel: w244 -> [w264 _]
            tunnel: w240 -> [w263 _]
            tunnel: w237 -> [_ w271]
            tunnel: w235 -> [_ w272]
            frame False {
              n90 = Less Or Equal To 0?(x=w263) -> (x <= 0?=w266:bool)
              n91 = Less Or Equal To 0?(x=w264) -> (x <= 0?=w265:bool)
              n92 = Or(x=w266, y=w265) -> (x .or. y?=w267:bool)
              n93 = case shown="False" w267 {
                tunnel: [u8 2 ("Det 3") _] -> w268
                frame False {
                }
                frame True {
                }
              }
            }
            frame True {
              n94 = Less Or Equal?(x=w272, y=w271) -> (x <= y?=w270:bool)
              n95 = case shown="True" w270 {
                tunnel: [_ u8 4 ("Det 3")] -> w273
                frame False {
                }
                frame True {
                }
              }
            }
          }
          n96 = Bundle By Name(cluster=T16 {"First Correlation"=0, "Latest Correlation"=0}, "First Correlation"=w241) -> (w250:T16)
        }
        frame 4 {
          # "This section ensures that we only look for the particle\nwithin the speed bounds of the current filter"
          n97 = Increment(x=w276) -> (x+1=w275:T15)
          n98 = Unbundle By Name(w282) -> ("Detector Max Speed Count"=w280:i32)
          n99 = Unbundle By Name(w275) -> ("First Detector Count"=w281:i32)
          n100 = Greater Or Equal?(x=w281, y=w280) -> (x >= y?=w279:bool)
          n101 = case shown="True" w279 {
            tunnel: [u8 5 u8 4] -> w278
            frame True {
            }
            frame False {
            }
          }
        }
        frame 5 {
          # "Waits for a reverse correlation that's close to the first correlation, but make sure it's in the right speed range."
          n102 = Unbundle By Name(w300) -> ("Detector Min Speed Count"=w299:i32)
          n103 = Unbundle By Name(w287) -> ("First Correlation"=w292:i32)
          n104 = Increment(x=w290) -> (x+1=w285:T15)
          n105 = Unbundle By Name(w285) -> ("First Detector Count"=w291:i32)
          n106 = Add(x=w295, y=w294) -> (x+y=w286:i32)
          n107 = Greater Or Equal?(x=w291, y=w299) -> (x >= y?=w298:bool)
          n108 = case shown="False" w298 {
            tunnel: [_ w316] -> w293
            tunnel: [u8 5 _] -> _
            tunnel: w297 -> [_ w315]
            tunnel: w296 -> [_ w312]
            tunnel: w292 -> [_ w303]
            tunnel: [_ w302] -> w288
            frame True {
            }
            frame False {
              n109 = Unbundle By Name(w312) -> ("Filter 1.Det 1"=w309:i32, "Filter 1.Det 1"=w311:i32, "Filter 1.Det 1"=w310:i32)
              n110 = To Fixed-Point(number=w303) -> (fixed-point=w305:fxp<+/-,32,32>)  [unwired: 1 in]
              n111 = Subtract(x=fxp<+,1,1> 1.0, y=w315) -> (x-y=w313:fxp<+,33,1>)
              n112 = Add(x=w311, y=w310) -> (x+y=w308:i32)
              n113 = Multiply(x=w313, y=w305) -> (x*y=w307:fxp<+/-,64,32>)
              n114 = Subtract(x=w309, y=w308) -> (x-y=w302:i32)
              n115 = To Fixed-Point(number=w302) -> (fixed-point=w304:fxp<+/-,32,32>)  [unwired: 1 in]
              n116 = Greater?(x=w304, y=w307) -> (0:w306:bool)
              n117 = case shown="True" w306 {
                tunnel: [u8 6 u8 5] -> w316
                frame True {
                }
                frame False {
                }
              }
            }
          }
          n118 = Bundle(cluster=w287, "Latest Correlation"=w288) -> (w289:T16)  [unwired: 1 in]
        }
        frame 6 {
          # "Waits for Boxcar 2 to reach the halfway point\nbetween Boxcars 1 and 3+4."
          n119 = Unbundle By Name(w328) -> ("Detector Min Speed Count"=w324:i32)
          n120 = Unbundle By Name(w344) -> ("Filter 1.Det 1"=w354:i32, "Filter 1.Det 1"=w357:i32, "Filter 1.Det 1"=w356:i32, "Filter 1.Det 1"=w348:i32)
          n121 = Unbundle By Name(w327) -> ("First Detector Count"=w325:i32)
          n122 = Increment(x=w327) -> (x+1=w338:T15)
          n123 = To Fixed-Point(number=w352) -> (fixed-point=w341:fxp<+/-,32,32>)  [unwired: 1 in]
          n124 = Decrement(x=w360) -> (x-1=w340:i32)
          n125 = Increment(x=w337) -> (x+1=w334:fxp<+,33,1>)
          n126 = Add(x=w357, y=w356) -> (x+y=w355:i32)
          n127 = Unbundle(w326) -> ("First Correlation"=w336:i32, "Latest Correlation"=w320:i32)
          n128 = To Fixed-Point(number=w336) -> (fixed-point=w335:fxp<+/-,32,32>)  [unwired: 1 in]
          n129 = Add(x=w354, y=w355) -> (x+y=w358:i32)
          n130 = Subtract(x=w354, y=w355) -> (x-y=w333:i32)
          n131 = To Fixed-Point(number=w348) -> (fixed-point=w343:fxp<+/-,32,32>)  [unwired: 1 in]
          n132 = Multiply(x=w335, y=w334) -> (x*y=w331:fxp<+/-,64,33>)
          n133 = To Fixed-Point(number=w351) -> (fixed-point=w342:fxp<+/-,32,32>)  [unwired: 1 in]
          n134 = To Fixed-Point(number=w358) -> (fixed-point=w345:fxp<+/-,32,32>)  [unwired: 1 in]
          n135 = Greater Or Equal?(x=w325, y=w324) -> (x >= y?=w323:bool)
          n136 = Multiply(x=w345, y=w341) -> (x*y=w353:fxp<+/-,64,64>)
          n137 = To Fixed-Point(number=w333) -> (fixed-point=w332:fxp<+/-,32,32>)  [unwired: 1 in]
          n138 = Scale By Power Of 2(n=i16 1, x=w342) -> (x*2^n=w349:fxp<+/-,32,32>)
          n139 = Max & Min(x=w333, y=w320) -> (max(x,y)=w319:i32)  [unwired: 1 out]
          n140 = Greater?(x=w332, y=w331) -> (0:w330:bool)
          n141 = Multiply(x=w343, y=w349) -> (x*y=w347:fxp<+/-,64,64>)
          n142 = Or(x=w330, y=w323) -> (x .or. y?=w329:bool)
          n143 = Less?(x=w353, y=w347) -> (x < y?=w339:bool)
          n144 = case shown="True" w339 {
            tunnel: [w365 u8 7 ("Det 3")] -> w359
            tunnel: w340 -> [w362 _]
            tunnel: w329 -> [w361 _]
            frame False {
              n145 = Less Or Equal To 0?(x=w362) -> (x <= 0?=w363:bool)
              n146 = Or(x=w361, y=w363) -> (x .or. y?=w364:bool)
              n147 = case shown="False" w364 {
                tunnel: [u8 6 ("Det 3") _] -> w365
                frame False {
                }
                frame True {
                  (unwired) u8 6 ("Det 3")
                }
              }
            }
            frame True {
            }
          }
          n148 = Bundle By Name(cluster=w326, "Latest Correlation"=w319) -> (w346:T16)
          n149 = Bundle By Name(cluster=w338, "Detector Gap Count"=0) -> (w322:T15)
        }
        frame 7 {
          # "q = ADC value / CSA sensitivity"
          # "Ensures the charge is good"
          n150 = Unbundle(w374) -> ("First Correlation"=w388:i32, "Latest Correlation"=w387:i32)
          n151 = Unbundle By Name(w389) -> ("High Charge Limit"=w368:fxp<+,32,-41>, "Low Charge Limit"=w385:fxp<+,32,-41>)
          n152 = Add(x=w388, y=w387) -> (x+y=w377:i32)
          n153 = Increment(x=w372) -> (x+1=w371:T15)
          n154 = Scale By Power Of 2(n=i16 -1, x=w377) -> (x*2^n=w375:i32)
          n155 = To Fixed-Point(number=w375) -> (fixed-point=w376:fxp<+/-,32,32>)  [unwired: 1 in]
          n156 = Multiply(x=w376, y=w386) -> (x*y=w380:fxp<+/-,47,32>)
          n157 = Multiply(x=w380, y=w379) -> (x*y=w370:fxp<+/-,64,-17>)
          n158 = Bundle(cluster=w374, "First Correlation"=w375) -> (w373:T16)  [unwired: 1 in]
          n159 = To Fixed-Point(fixed-point type=w368, number=w370) -> (fixed-point=w369:fxp<+,32,-41>)
          n160 = Less Or Equal?(x=w369, y=w368) -> (x <= y?=w384:bool)
          n161 = Greater Or Equal?(x=w369, y=w385) -> (x >= y?=w383:bool)
          n162 = And(x=w384, y=w383) -> (x .and. y?=w382:bool)
          n163 = case shown="True" w382 {
            tunnel: [u8 8 ("Det 3") _] -> w381
            frame True {
            }
            frame False {
              (unwired) u8 7 ("Det 3")
            }
          }
        }
        frame 8 {
          # "This section ensures that we only look for the particle\nwithin the speed bounds of the current filter"
          n164 = Increment(x=w393) -> (x+1=w392:T15)
          n165 = Unbundle By Name(w399) -> ("Gap Max Speed Count"=w397:i32)
          n166 = Unbundle By Name(w392) -> ("Detector Gap Count"=w398:i32)
          n167 = Greater Or Equal?(x=w398, y=w397) -> (x >= y?=w396:bool)
          n168 = case shown="True" w396 {
            tunnel: [u8 9 u8 8] -> w395
            frame True {
            }
            frame False {
            }
          }
        }
        frame 9 {
          # "Waits for a second detector correlation that's close to the\nfirst correlation, but make sure it's in the right speed range."
          n169 = Unbundle By Name(w405) -> ("First Correlation"=w408:i32)
          n170 = Increment(x=w406) -> (x+1=w403:T15)
          n171 = Unbundle By Name(w416) -> ("Gap Min Speed Count"=w415:i32)
          n172 = Unbundle By Name(w403) -> ("Detector Gap Count"=w407:i32)
          n173 = Add(x=w411, y=w410) -> (x+y=w404:i32)
          n174 = Greater Or Equal?(x=w407, y=w415) -> (x >= y?=w414:bool)
          n175 = case shown="False" w414 {
            tunnel: [_ w431] -> w409
            tunnel: w413 -> [_ w430]
            tunnel: w412 -> [_ w427]
            tunnel: w408 -> [_ w418]
            frame True {
              (unwired) u8 9
            }
            frame False {
              n176 = Unbundle By Name(w427) -> ("Filter 1.Det 1"=w424:i32, "Filter 1.Det 1"=w426:i32, "Filter 1.Det 1"=w425:i32)
              n177 = To Fixed-Point(number=w418) -> (fixed-point=w420:fxp<+/-,32,32>)  [unwired: 1 in]
              n178 = Subtract(x=fxp<+,1,1> 1.0, y=w430) -> (x-y=w428:fxp<+,33,1>)
              n179 = Add(x=w426, y=w425) -> (x+y=w423:i32)
              n180 = Multiply(x=w428, y=w420) -> (x*y=w422:fxp<+/-,64,32>)
              n181 = Subtract(x=w423, y=w424) -> (x-y=w417:i32)
              n182 = To Fixed-Point(number=w417) -> (fixed-point=w419:fxp<+/-,32,32>)  [unwired: 1 in]
              n183 = Greater?(x=w419, y=w422) -> (0:w421:bool)
              n184 = case shown="True" w421 {
                tunnel: [u8 10 u8 9] -> w431
                frame True {
                }
                frame False {
                }
              }
            }
          }
        }
        frame 10 {
          # "Waits for Boxcar 2 to reach the halfway point\nbetween Boxcars 1 and 3+4."
          n185 = Unbundle By Name(w458) -> ("Filter 1.Det 2"=w467:i32, "Filter 1.Det 2"=w470:i32, "Filter 1.Det 2"=w469:i32, "Filter 1.Det 2"=w461:i32)
          n186 = Increment(x=w442) -> (x+1=w437:T15)
          n187 = To Fixed-Point(number=w465) -> (fixed-point=w455:fxp<+/-,32,32>)  [unwired: 1 in]
          n188 = Unbundle By Name(w441) -> ("Gap Min Speed Count"=w439:i32)
          n189 = Unbundle By Name(w442) -> ("Detector Gap Count"=w440:i32)
          n190 = Decrement(x=w473) -> (x-1=w454:i32)
          n191 = Increment(x=w452) -> (x+1=w448:fxp<+,33,1>)
          n192 = Add(x=w470, y=w469) -> (x+y=w468:i32)
          n193 = Unbundle(w451) -> ("First Correlation"=w450:i32)  [unwired: 1 out]
          n194 = To Fixed-Point(number=w450) -> (fixed-point=w449:fxp<+/-,32,32>)  [unwired: 1 in]
          n195 = Add(x=w467, y=w468) -> (x+y=w471:i32)
          n196 = Subtract(x=w468, y=w467) -> (x-y=w447:i32)
          n197 = To Fixed-Point(number=w461) -> (fixed-point=w457:fxp<+/-,32,32>)  [unwired: 1 in]
          n198 = Multiply(x=w449, y=w448) -> (x*y=w445:fxp<+/-,64,33>)
          n199 = To Fixed-Point(number=w464) -> (fixed-point=w456:fxp<+/-,32,32>)  [unwired: 1 in]
          n200 = To Fixed-Point(number=w471) -> (fixed-point=w459:fxp<+/-,32,32>)  [unwired: 1 in]
          n201 = Multiply(x=w459, y=w455) -> (x*y=w466:fxp<+/-,64,64>)
          n202 = To Fixed-Point(number=w447) -> (fixed-point=w446:fxp<+/-,32,32>)  [unwired: 1 in]
          n203 = Scale By Power Of 2(n=i16 1, x=w456) -> (x*2^n=w462:fxp<+/-,32,32>)
          n204 = Greater Or Equal?(x=w440, y=w439) -> (x >= y?=w438:bool)
          n205 = Greater?(x=w446, y=w445) -> (0:w444:bool)
          n206 = Multiply(x=w457, y=w462) -> (x*y=w460:fxp<+/-,64,64>)
          n207 = Or(x=w444, y=w438) -> (x .or. y?=w443:bool)
          n208 = Greater?(x=w466, y=w460) -> (0:w453:bool)
          n209 = case shown="True" w453 {
            tunnel: [w478 u8 11 ("Det 3")] -> w472
            tunnel: w454 -> [w475 _]
            tunnel: w443 -> [w474 _]
            frame False {
              n210 = Less Or Equal To 0?(x=w475) -> (x <= 0?=w476:bool)
              n211 = Or(x=w474, y=w476) -> (x .or. y?=w477:bool)
              n212 = case shown="False" w477 {
                tunnel: [u8 10 ("Det 3") _] -> w478
                frame False {
                }
                frame True {
                  (unwired) u8 10 ("Det 3")
                }
              }
            }
            frame True {
            }
          }
          n213 = Bundle By Name(cluster=w437, "Second Detector Count"=0) -> (w436:T15)
        }
        frame 11 {
          # "This section ensures that we only look for the particle\nwithin the speed bounds of the current filter"
          n214 = Increment(x=w483) -> (x+1=w482:T15)
          n215 = Unbundle By Name(w489) -> ("Detector Max Speed Count"=w487:i32)
          n216 = Unbundle By Name(w482) -> ("Second Detector Count"=w488:i32)
          n217 = Greater Or Equal?(x=w488, y=w487) -> (x >= y?=w486:bool)
          n218 = case shown="True" w486 {
            tunnel: [u8 12 u8 11] -> w485
            frame True {
            }
            frame False {
            }
          }
        }
        frame 12 {
          # "Waits for a reverse correlation that's close to the first correlation, but make sure it's in the right speed range."
          n219 = Unbundle By Name(w506) -> ("Detector Min Speed Count"=w505:i32)
          n220 = Unbundle By Name(w492) -> ("First Correlation"=w498:i32)
          n221 = Increment(x=w496) -> (x+1=w494:T15)
          n222 = Unbundle By Name(w494) -> ("Second Detector Count"=w497:i32)
          n223 = Add(x=w501, y=w500) -> (x+y=w495:i32)
          n224 = Greater Or Equal?(x=w497, y=w505) -> (x >= y?=w504:bool)
          n225 = case shown="False" w504 {
            tunnel: [_ w521] -> w499
            tunnel: w503 -> [_ w520]
            tunnel: w502 -> [_ w517]
            tunnel: w498 -> [_ w508]
            frame True {
              (unwired) u8 12
            }
            frame False {
              n226 = Unbundle By Name(w517) -> ("Filter 1.Det 2"=w514:i32, "Filter 1.Det 2"=w516:i32, "Filter 1.Det 2"=w515:i32)
              n227 = To Fixed-Point(number=w508) -> (fixed-point=w510:fxp<+/-,32,32>)  [unwired: 1 in]
              n228 = Subtract(x=fxp<+,1,1> 1.0, y=w520) -> (x-y=w518:fxp<+,33,1>)
              n229 = Add(x=w516, y=w515) -> (x+y=w513:i32)
              n230 = Multiply(x=w518, y=w510) -> (x*y=w512:fxp<+/-,64,32>)
              n231 = Subtract(x=w514, y=w513) -> (x-y=w507:i32)
              n232 = To Fixed-Point(number=w507) -> (fixed-point=w509:fxp<+/-,32,32>)  [unwired: 1 in]
              n233 = Greater?(x=w509, y=w512) -> (0:w511:bool)
              n234 = case shown="True" w511 {
                tunnel: [u8 13 u8 12] -> w521
                frame True {
                }
                frame False {
                }
              }
            }
          }
        }
        frame 13 {
          # "Waits for Boxcar 2 to reach the halfway point\nbetween Boxcars 1 and 3+4."
          n235 = Unbundle By Name(w531) -> ("Detector Min Speed Count"=w528:i32)
          n236 = Unbundle By Name(w546) -> ("Filter 1.Det 2"=w555:i32, "Filter 1.Det 2"=w558:i32, "Filter 1.Det 2"=w557:i32, "Filter 1.Det 2"=w549:i32)
          n237 = Unbundle By Name(w530) -> ("Second Detector Count"=w529:i32)
          n238 = Increment(x=w530) -> (x+1=w540:T15)
          n239 = To Fixed-Point(number=w553) -> (fixed-point=w543:fxp<+/-,32,32>)  [unwired: 1 in]
          n240 = Decrement(x=w561) -> (x-1=w542:i32)
          n241 = Increment(x=w539) -> (x+1=w536:fxp<+,33,1>)
          n242 = Add(x=w558, y=w557) -> (x+y=w556:i32)
          n243 = Unbundle(w524) -> ("First Correlation"=w538:i32)  [unwired: 1 out]
          n244 = To Fixed-Point(number=w538) -> (fixed-point=w537:fxp<+/-,32,32>)  [unwired: 1 in]
          n245 = Add(x=w555, y=w556) -> (x+y=w559:i32)
          n246 = Subtract(x=w555, y=w556) -> (x-y=w535:i32)
          n247 = To Fixed-Point(number=w549) -> (fixed-point=w545:fxp<+/-,32,32>)  [unwired: 1 in]
          n248 = Multiply(x=w537, y=w536) -> (x*y=w533:fxp<+/-,64,33>)
          n249 = To Fixed-Point(number=w552) -> (fixed-point=w544:fxp<+/-,32,32>)  [unwired: 1 in]
          n250 = To Fixed-Point(number=w559) -> (fixed-point=w547:fxp<+/-,32,32>)  [unwired: 1 in]
          n251 = Greater Or Equal?(x=w529, y=w528) -> (x >= y?=w526:bool)
          n252 = Multiply(x=w547, y=w543) -> (x*y=w554:fxp<+/-,64,64>)
          n253 = To Fixed-Point(number=w535) -> (fixed-point=w534:fxp<+/-,32,32>)  [unwired: 1 in]
          n254 = Scale By Power Of 2(n=i16 1, x=w544) -> (x*2^n=w550:fxp<+/-,32,32>)
          n255 = Greater?(x=w534, y=w533) -> (0:w532:bool)
          n256 = Multiply(x=w545, y=w550) -> (x*y=w548:fxp<+/-,64,64>)
          n257 = Or(x=w532, y=w526) -> (x .or. y?=w527:bool)
          n258 = Less?(x=w554, y=w548) -> (x < y?=w541:bool)
          n259 = case shown="True" w541 {
            tunnel: [w566 u8 14 ("Det 3")] -> w560
            tunnel: w542 -> [w563 _]
            tunnel: w527 -> [w562 _]
            frame False {
              n260 = Less Or Equal To 0?(x=w563) -> (x <= 0?=w564:bool)
              n261 = Or(x=w562, y=w564) -> (x .or. y?=w565:bool)
              n262 = case shown="False" w565 {
                tunnel: [u8 13 ("Det 3") _] -> w566
                frame False {
                }
                frame True {
                  (unwired) u8 13 ("Det 3")
                }
              }
            }
            frame True {
            }
          }
        }
        frame 14 {
          # "Look carefully at the way the Armed variable is treated in here.\nIf One Shot implies Armed (ie, it's okay to let a particle through),\nthe particle is allowed to go through, but Armed is turned off."
          # "v = clockspeed * distance / speed count"
          # "1/2mv^2 = Vq\ntherefore\nm = 2Vq/v^2"
          n263 = Unbundle By Name(w570) -> ("First Detector Count"=w569:i32)
          n264 = Unbundle By Name(w598) -> ("High Velocity Limit"=w585:fxp<+,18,18>, "Low Velocity Limit"=w586:fxp<+,18,18>, "High Mass Limit"=w594:fxp<+,32,-37>, "Low Mass Limit"=w574:fxp<+,32,-37>, "High Voltage"=w589:fxp<+,32,22>)
          n265 = Multiply(x=w589, y=w576) -> (x*y=w595:fxp<+,64,-19>)
          n266 = To Fixed-Point(number=w569) -> (fixed-point=w584:fxp<+/-,32,32>)  [unwired: 1 in]
          n267 = To Fixed-Point(number=w569) -> (fixed-point=w577:fxp<+/-,32,32>)  [unwired: 1 in]
          n268 = Square(x=w577) -> (x^2=w578:fxp<+,63,63>)
          n269 = Multiply(x=w585, y=w584) -> (x*y=w583:fxp<+/-,50,50>)
          n270 = Multiply(x=w584, y=w586) -> (x*y=w582:fxp<+/-,50,50>)
          n271 = Multiply(x=w597, y=w578) -> (x*y=w596:fxp<+,64,19>)
          n272 = To Fixed-Point(fixed-point type=fxp<+,32,-13> 0.0, number=w596) -> (fixed-point=w572:fxp<+,32,-13>)
          n273 = Greater Or Equal?(x=w583, y=w575) -> (x >= y?=w593:bool)
          n274 = Less Or Equal?(x=w582, y=w575) -> (x <= y?=w592:bool)
          n275 = Multiply(x=w595, y=w572) -> (x*y=w579:fxp<+,64,-32>)
          n276 = Scale By Power Of 2(n=i16 1, x=w579) -> (x*2^n=w573:fxp<+,64,-32>)
          n277 = Less Or Equal?(x=w573, y=w594) -> (x <= y?=w591:bool)
          n278 = Greater Or Equal?(x=w573, y=w574) -> (x >= y?=w590:bool)
          n279 = Compound Arithmetic op=AND(w593, w592, w591, w590, w581) -> (w580:bool)
          n280 = case shown="True" w580 {
            tunnel: [u8 15 ("Det 3") _] -> w587
            frame True {
            }
            frame False {
              (unwired) u8 14 ("Det 3")
            }
          }
        }
        frame 15 {
          # "To keep the names in the distance cluster from\ncorrupting the names of the speed counts cluster.\nThis really shouldn't happen, but it does."
          n281 = Unbundle By Name(w609) -> ("First Detector Count"=w615:i32)
          n282 = To Fixed-Point(number=w615) -> (fixed-point=w623:fxp<+/-,32,32>)  [unwired: 1 in]
          n283 = Multiply(x=w623, y=w622) -> (x*y=w621:T20)
          n284 = To Long Integer(number=w621) -> (32bit integer=w620:T21)
          n285 = Scale By Power Of 2(n=i16 -1, x=w613) -> (x*2^n=w614:i32)
          n286 = Subtract(x=w620, y=w619) -> (x-y=w618:T21)
          n287 = Subtract(x=w618, y=w614) -> (x-y=w611:T21)
          n288 = Unbundle By Name(w611) -> ("Distance to PSU"=w608:i32, "Distance to end of PSU"=w607:i32, "Distance to DCS 2"=w606:i32, "Distance to front of LEIL Chamber"=w602:i32, "Distance to DCS 1"=w600:i32)
          n289 = To Long Integer(number=w602) -> (32bit integer=w601:i32)
          n290 = To Long Integer(number=w608) -> (32bit integer=w605:i32)
          n291 = To Long Integer(number=w607) -> (32bit integer=w604:i32)
          n292 = To Long Integer(number=w606) -> (32bit integer=w603:i32)
          n293 = Add(x=w600, y=w616) -> ()  [unwired: 1 out]
          n294 = Bundle(cluster=w609, "First Detector Count"=w605, "Detector Gap Count"=w604, "Second Detector Count"=w603, "Second Detector Final Count"=w601) -> (w610:T15)
        }
        frame 16 {
          n295 = Decrement(x=w650) -> (x-1=w649:T15)
          n296 = Decrement(x=w632) -> (x-1=w625:i32)
          n297 = Unbundle(w649) -> ("First Detector Count"=w646:i32, "Detector Gap Count"=w644:i32, "Second Detector Count"=w641:i32, "Second Detector Final Count"=w639:i32)
          n298 = Add(x=w641, y=w629) -> (x+y=w642:i32)
          n299 = Add(x=w639, y=w629) -> (x+y=w628:i32)
          n300 = Add(x=w625, y=w629) -> (x+y=w627:i32)
          n301 = Less Or Equal To 0?(x=w641) -> (x <= 0?=w640:bool)
          n302 = Greater Or Equal To 0?(x=w628) -> (x >= 0?=w637:bool)
          n303 = Greater Or Equal To 0?(x=w627) -> (x >= 0?=w624:bool)
          n304 = Less Or Equal To 0?(x=w646) -> (x <= 0?=w645:bool)
          n305 = Less Or Equal To 0?(x=w639) -> (x <= 0?=w638:bool)
          n306 = Less Or Equal To 0?(x=w625) -> (x <= 0?=w626:bool)
          n307 = Greater Or Equal To 0?(x=w642) -> (x >= 0?=w634:bool)
          n308 = Greater Or Equal To 0?(x=w644) -> (x >= 0?=w643:bool)
          n309 = And(x=w638, y=w637) -> (x .and. y?=w631:bool)
          n310 = And(x=w626, y=w624) -> (x .and. y?=w630:bool)
          n311 = And(x=w645, y=w643) -> (x .and. y?=w648:bool)
          n312 = And(x=w640, y=w634) -> (x .and. y?=w647:bool)
          n313 = And(x=w633, y=w637) -> (x .and. y?=w635:bool)
          n314 = Compound Arithmetic op=OR(w635, w634, w624) -> (w636:bool)
          n315 = case shown="False" w636 {
            tunnel: [u8 16 ("Det 3") _] -> w651
            frame True {
            }
            frame False {
            }
          }
        }
      }
    }
    n316 = Delete From Array(array=w90) -> (array with subset deleted=w89:cluster{"Det 1":i16, "Det 2":i16}[])  [unwired: 2 in, 1 out]
    n317 = case shown="True" "Calibrate" {
      tunnel: w99 -> [w156 _]
      tunnel: [w156 w157] -> w132
      tunnel: w85 -> [_ w157]
      frame False {
      }
      frame True {
      }
    }
    n318 = Or Array Elements(Boolean array=w109) -> (logical OR=w103:bool)
    n319 = Or Array Elements(Boolean array=w71) -> (logical OR=w77:bool)
    n320 = Or Array Elements(Boolean array=w112) -> (logical OR=w84:bool)
    n321 = Or Array Elements(Boolean array=w111) -> (logical OR=w81:bool)
    n322 = Or Array Elements(Boolean array=w110) -> (logical OR=w79:bool)
    n323 = Not(x=w103) -> (.not. x?=w108:bool)
    n324 = And(x=w108, y=w106) -> (x .and. y?=w107:bool)
    n325 = xnode ("Handshake Write")("Data"=w79, "Input Valid"=TRUE) -> ()  [unwired: 1 in, 2 out]
    n326 = xnode ("Handshake Write")("Data"=w84, "Input Valid"=TRUE) -> ()  [unwired: 1 in, 2 out]
    n327 = local write "Armed"(w107) -> ()
    n328 = xnode ("Handshake Write")("Data"=w81, "Input Valid"=TRUE) -> ()  [unwired: 1 in, 2 out]
    n329 = xnode ("Handshake Write")("Data"=w77, "Input Valid"=TRUE) -> ()  [unwired: 1 in, 2 out]
  }
  n330 = node-c288(w38) -> ()
  n331 = node-c288(w24) -> ()
